vi "Spreadsheet String to Array Variant.vi"(8 "error in (no error)":errorcluster, 10 "spreadsheet string in":string, 11 "Array Variant in (type)":variant) -> (0 "error out":errorcluster, 3 "Array Variant out":variant)   [LabVIEW 2020, in "Generic Config Handling.lvlib"]
doc: "This vi converts a spreadsheet string into a variant which represents an array. The variant in is used to get the type."
uses:
  Generic Config Handling.lvlib
  <vilib>/Utility/VariantDataType/VariantType.lvlib
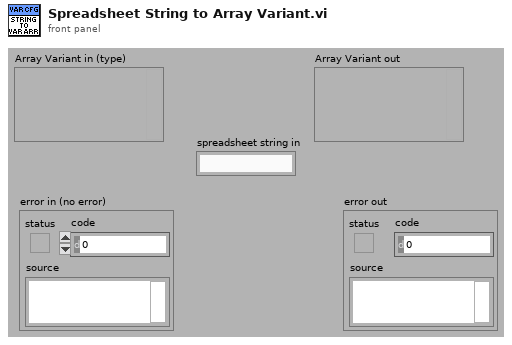
[diagram p1: front panel]
types:
  T1 = typedef "VariantType.lvlib/Type.ctl" = enum8{"Invalid Type", "Void", "I8", "I16", "I32", "I64", "U8", "U16", "U32", "U64", "Single Float", "Double Float", "Extended Float", "Single Complex", "Double Complex", "Extended Complex", "Enum U8", "Enum U16", "Enum U32", "Enum U64", "Single Float With Unit", "Double Float With Unit", "Extended Float With Unit", "Single Complex with Unit", "Double Complex with Unit", "Extended Complex with Unit", "Boolean", "String", "Path", "Picture", "Tag", "Array", "Cluster", "Variant", "LV Variant", "Waveform", "Timestamp", "Digital Waveform", "Digital Data", "ExpressData", "Refnum", "External Data", "VI", "Poly VI", "LabVIEW Class Instance", "Fixed Point"}
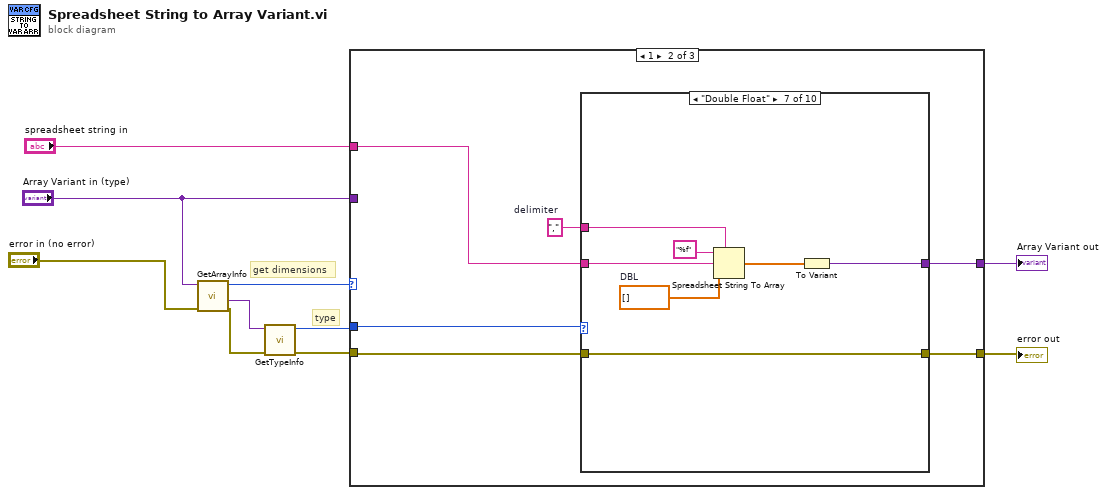
[diagram p0: block diagram]
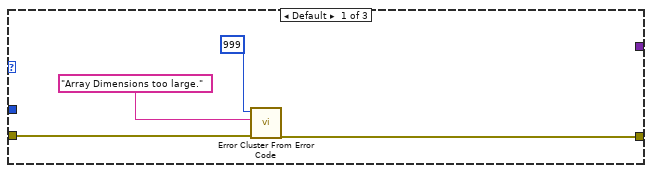
[diagram p2: hidden frame]
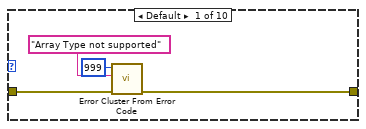
[diagram p3: hidden frame]
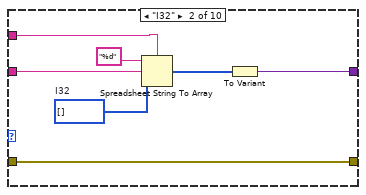
[diagram p4: hidden frame]
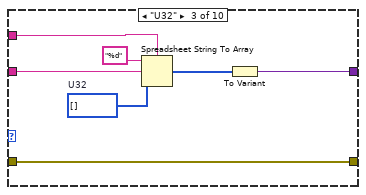
[diagram p5: hidden frame]
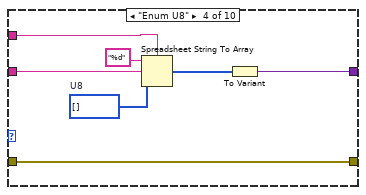
[diagram p6: hidden frame]
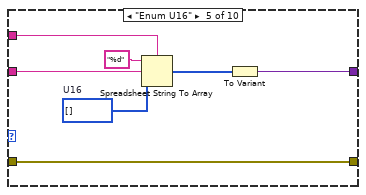
[diagram p7: hidden frame]
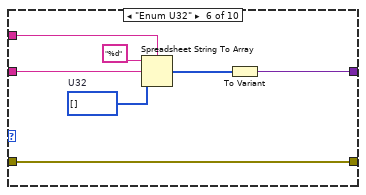
[diagram p8: hidden frame]
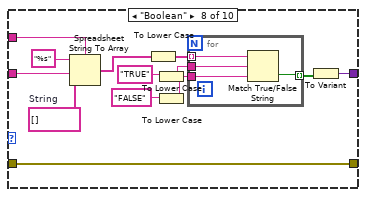
[diagram p9: hidden frame]
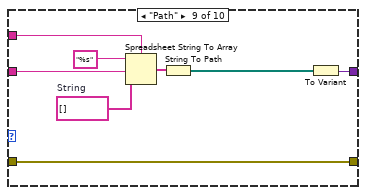
[diagram p10: hidden frame]
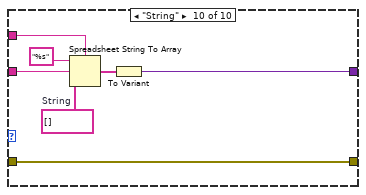
[diagram p11: hidden frame]
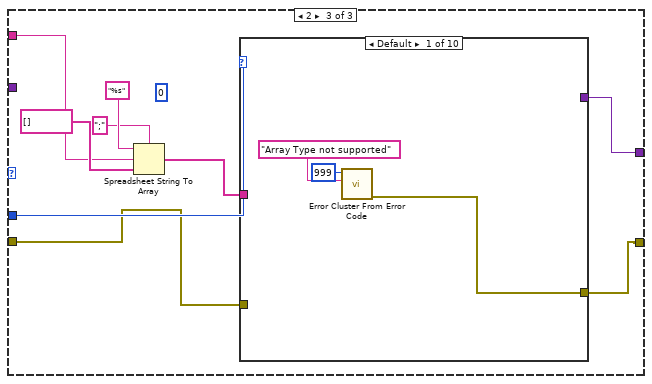
[diagram p12: hidden frame]
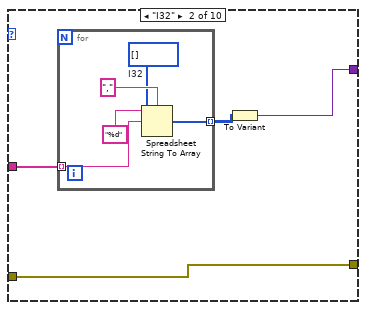
[diagram p13: hidden frame]
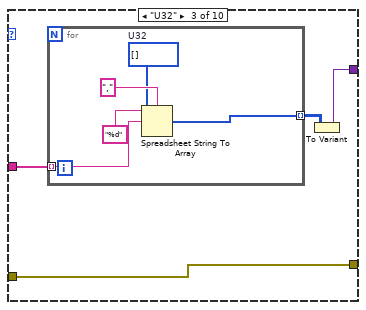
[diagram p14: hidden frame]
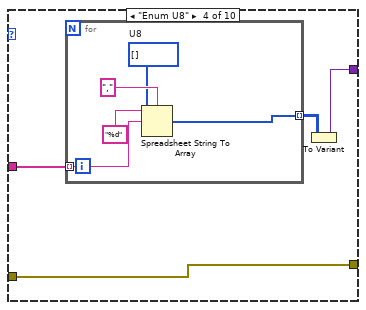
[diagram p15: hidden frame]
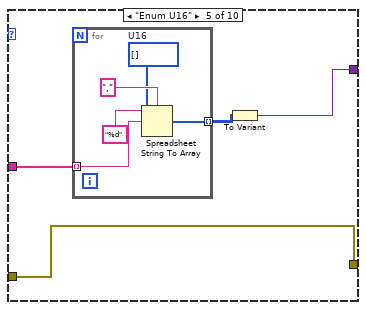
[diagram p16: hidden frame]
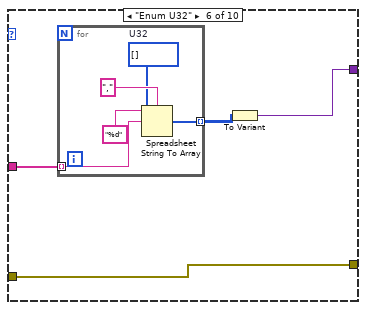
[diagram p17: hidden frame]
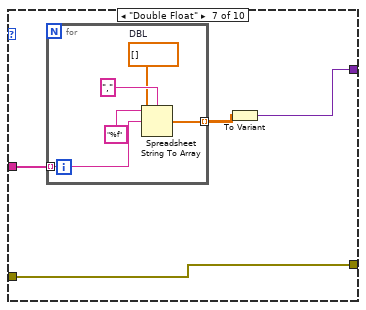
[diagram p18: hidden frame]
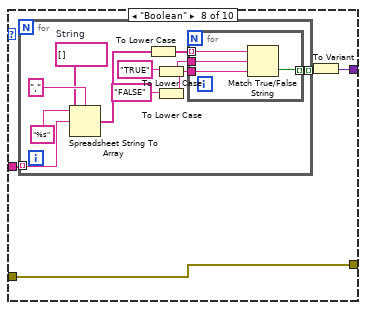
[diagram p19: hidden frame]
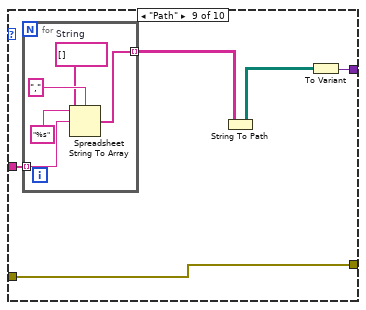
[diagram p20: hidden frame]
diagram:
  # "type"
  # "get dimensions"
  n1 = call <vilib>:"GetArrayInfo.vi"("error in (no error)"="error in (no error)", "Variant"="Array Variant in (type)") -> ("error out"=w7:errorcluster, "ArrayElement"=w6:variant, "NDims"=w4:i32)  [unwired: 6 in, 1 out]
  n2 = call <vilib>:"GetTypeInfo.vi"("error in (no error)"=w7, "Variant"=w6) -> ("error out"=w10:errorcluster, "Type Enum"=w8:T1)  [unwired: 5 in, 3 out]
  n3 = case shown="1" w4 {
    tunnel: w10 -> [w12 w18 w105]
    tunnel: [w11 w19 w106] -> w3
    tunnel: "Array Variant in (type)" -> [_ _ _]
    tunnel: w8 -> [_ w20 w107]
    tunnel: "spreadsheet string in" -> [_ w17 w100]
    tunnel: [_ w16 w104] -> w1
    frame Default {
      n4 = call <vilib>:"Error Cluster From Error Code.vi"("error in (no error)"=w12, "error message (\"\")"="Array Dimensions too large." ("error message (\"\")"), "error code (0)"=999) -> ("error out"=w11:errorcluster)  [unwired: 6 in]
    }
    frame 1 {
      w15 = ","  # delimiter
      n5 = case shown="\"Double Float\"" w20 {
        tunnel: [w22 w26 w33 w40 w47 w54 w61 w75 w87 w94] -> w19
        tunnel: w18 -> [w21 w26 w33 w40 w47 w54 w61 w75 w87 w94]
        tunnel: w17 -> [_ w31 w38 w45 w52 w59 w66 w79 w91 w98]
        tunnel: [_ w27 w34 w41 w48 w55 w62 w76 w88 w95] -> w16
        tunnel: w15 -> [_ w25 w32 w39 w46 w53 w60 w67 w84 w92]
        frame Default {
          n6 = call <vilib>:"Error Cluster From Error Code.vi"("error in (no error)"=w21, "error message (\"\")"="Array Type not supported" ("error message (\"\")"), "error code (0)"=999) -> ("error out"=w22:errorcluster)  [unwired: 6 in]
        }
        frame "I32" {
          w29 = i32[] []  # I32
          n7 = Spreadsheet String To Array(delimiter (Tab)=w25, format string="%d", spreadsheet string=w31, array type (2D Dbl)=w29) -> (array=w28:i32[])
          n8 = To Variant(anything=w28) -> (Variant=w27:variant)
        }
        frame "U32" {
          w36 = u32[] []  # U32
          n9 = Spreadsheet String To Array(delimiter (Tab)=w32, format string="%d", spreadsheet string=w38, array type (2D Dbl)=w36) -> (array=w35:u32[])
          n10 = To Variant(anything=w35) -> (Variant=w34:variant)
        }
        frame "Enum U8" {
          w43 = u8[] []  # U8
          n11 = Spreadsheet String To Array(delimiter (Tab)=w39, format string="%d", spreadsheet string=w45, array type (2D Dbl)=w43) -> (array=w42:u8[])
          n12 = To Variant(anything=w42) -> (Variant=w41:variant)
        }
        frame "Enum U16" {
          w50 = u16[] []  # U16
          n13 = Spreadsheet String To Array(delimiter (Tab)=w46, format string="%d", spreadsheet string=w52, array type (2D Dbl)=w50) -> (array=w49:u16[])
          n14 = To Variant(anything=w49) -> (Variant=w48:variant)
        }
        frame "Enum U32" {
          w57 = u32[] []  # U32
          n15 = Spreadsheet String To Array(delimiter (Tab)=w53, format string="%d", spreadsheet string=w59, array type (2D Dbl)=w57) -> (array=w56:u32[])
          n16 = To Variant(anything=w56) -> (Variant=w55:variant)
        }
        frame "Double Float" {
          w64 = dbl[] []  # DBL
          n17 = Spreadsheet String To Array(delimiter (Tab)=w60, format string="%f", spreadsheet string=w66, array type (2D Dbl)=w64) -> (array=w63:dbl[])
          n18 = To Variant(anything=w63) -> (Variant=w62:variant)
        }
        frame "Boolean" {
          w77 = string[] []  # String
          n19 = Spreadsheet String To Array(delimiter (Tab)=w67, format string="%s", spreadsheet string=w79, array type (2D Dbl)=w77) -> (array=w69:string[])
          n20 = To Lower Case(string=w69) -> (all lower case string=w74:string[])
          n21 = To Lower Case(string="TRUE" ("true string")) -> (all lower case string=w70:string)
          n22 = To Lower Case(string="FALSE" ("false string")) -> (all lower case string=w71:string)
          n23 = for {
            tunnel: w74 -> [w83] mode=indexing
            tunnel: w71 -> [w82]
            tunnel: w70 -> [w81]
            tunnel: [w80] -> w68 mode=indexing
            n24 = Match True/False String(2:w82, 3:w81, 4:w83) -> (0:w80:bool)  [unwired: 1 out]
          }
          n25 = To Variant(anything=w68) -> (Variant=w76:variant)
        }
        frame "Path" {
          w89 = string[] []  # String
          n26 = Spreadsheet String To Array(delimiter (Tab)=w84, format string="%s", spreadsheet string=w91, array type (2D Dbl)=w89) -> (array=w85:string[])
          n27 = String To Path(string=w85) -> (path=w86:path[])
          n28 = To Variant(anything=w86) -> (Variant=w88:variant)
        }
        frame "String" {
          w96 = string[] []  # String
          n29 = Spreadsheet String To Array(delimiter (Tab)=w92, format string="%s", spreadsheet string=w98, array type (2D Dbl)=w96) -> (array=w93:string[])
          n30 = To Variant(anything=w93) -> (Variant=w95:variant)
        }
      }
    }
    frame 2 {
      (unwired) u16 0
      n31 = Spreadsheet String To Array(delimiter (Tab)=";", format string="%s", spreadsheet string=w100, array type (2D Dbl)=string[] []) -> (array=w99:string[])
      n32 = case shown="Default" w107 {
        tunnel: [w108 w111 w122 w131 w138 w147 w156 w166 w186 w195] -> w106
        tunnel: w105 -> [_ w111 w122 w131 w138 w147 w156 w166 w186 w195]
        tunnel: w99 -> [_ w114 w123 w132 w141 w150 w159 w168 w188 w197]
        tunnel: [_ w112 w120 w129 w139 w148 w157 w167 w187 w196] -> w104
        frame Default {
          n33 = call <vilib>:"Error Cluster From Error Code.vi"("error message (\"\")"="Array Type not supported" ("error message (\"\")"), "error code (0)"=999) -> ("error out"=w108:errorcluster)  [unwired: 7 in]
        }
        frame "I32" {
          n34 = for {
            tunnel: w114 -> [w119] mode=indexing
            tunnel: [w115] -> w113 mode=indexing
            w116 = i32[] []  # I32
            n35 = Spreadsheet String To Array(delimiter (Tab)=",", format string="%d", spreadsheet string=w119, array type (2D Dbl)=w116) -> (array=w115:i32[])
          }
          n36 = To Variant(anything=w113) -> (Variant=w112:variant)
        }
        frame "U32" {
          n37 = for {
            tunnel: w123 -> [w128] mode=indexing
            tunnel: [w124] -> w121 mode=indexing
            w125 = u32[] []  # U32
            n38 = Spreadsheet String To Array(delimiter (Tab)=",", format string="%d", spreadsheet string=w128, array type (2D Dbl)=w125) -> (array=w124:u32[])
          }
          n39 = To Variant(anything=w121) -> (Variant=w120:variant)
        }
        frame "Enum U8" {
          n40 = for {
            tunnel: w132 -> [w137] mode=indexing
            tunnel: [w133] -> w130 mode=indexing
            w134 = u8[] []  # U8
            n41 = Spreadsheet String To Array(delimiter (Tab)=",", format string="%d", spreadsheet string=w137, array type (2D Dbl)=w134) -> (array=w133:u8[])
          }
          n42 = To Variant(anything=w130) -> (Variant=w129:variant)
        }
        frame "Enum U16" {
          n43 = for {
            tunnel: w141 -> [w146] mode=indexing
            tunnel: [w142] -> w140 mode=indexing
            w143 = u16[] []  # U16
            n44 = Spreadsheet String To Array(delimiter (Tab)=",", format string="%d", spreadsheet string=w146, array type (2D Dbl)=w143) -> (array=w142:u16[])
          }
          n45 = To Variant(anything=w140) -> (Variant=w139:variant)
        }
        frame "Enum U32" {
          n46 = for {
            tunnel: w150 -> [w155] mode=indexing
            tunnel: [w151] -> w149 mode=indexing
            w152 = u32[] []  # U32
            n47 = Spreadsheet String To Array(delimiter (Tab)=",", format string="%d", spreadsheet string=w155, array type (2D Dbl)=w152) -> (array=w151:u32[])
          }
          n48 = To Variant(anything=w149) -> (Variant=w148:variant)
        }
        frame "Double Float" {
          n49 = for {
            tunnel: w159 -> [w164] mode=indexing
            tunnel: [w160] -> w158 mode=indexing
            w161 = dbl[] []  # DBL
            n50 = Spreadsheet String To Array(delimiter (Tab)=",", format string="%f", spreadsheet string=w164, array type (2D Dbl)=w161) -> (array=w160:dbl[])
          }
          n51 = To Variant(anything=w158) -> (Variant=w157:variant)
        }
        frame "Boolean" {
          n52 = for {
            tunnel: w168 -> [w179] mode=indexing
            tunnel: [w169] -> w165 mode=indexing
            w176 = string[] []  # String
            n53 = Spreadsheet String To Array(delimiter (Tab)=",", format string="%s", spreadsheet string=w179, array type (2D Dbl)=w176) -> (array=w170:string[])
            n54 = To Lower Case(string=w170) -> (all lower case string=w175:string[])
            n55 = To Lower Case(string="TRUE" ("true string")) -> (all lower case string=w171:string)
            n56 = To Lower Case(string="FALSE" ("false string")) -> (all lower case string=w172:string)
            n57 = for {
              tunnel: w175 -> [w183] mode=indexing
              tunnel: w172 -> [w182]
              tunnel: w171 -> [w181]
              tunnel: [w180] -> w169 mode=indexing
              n58 = Match True/False String(2:w182, 3:w181, 4:w183) -> (0:w180:bool)  [unwired: 1 out]
            }
          }
          n59 = To Variant(anything=w165) -> (Variant=w167:variant)
        }
        frame "Path" {
          n60 = for {
            tunnel: w188 -> [w193] mode=indexing
            tunnel: [w189] -> w185 mode=indexing
            w190 = string[] []  # String
            n61 = Spreadsheet String To Array(delimiter (Tab)=",", format string="%s", spreadsheet string=w193, array type (2D Dbl)=w190) -> (array=w189:string[])
          }
          n62 = String To Path(string=w185) -> (path=w184:path[][])
          n63 = To Variant(anything=w184) -> (Variant=w187:variant)
        }
        frame "String" {
          n64 = for {
            tunnel: w197 -> [w202] mode=indexing
            tunnel: [w198] -> w194 mode=indexing
            w199 = string[] []  # String
            n65 = Spreadsheet String To Array(delimiter (Tab)=",", format string="%s", spreadsheet string=w202, array type (2D Dbl)=w199) -> (array=w198:string[])
          }
          n66 = To Variant(anything=w194) -> (Variant=w196:variant)
        }
      }
    }
  }
  "error out" <- w3
  "Array Variant out" <- w1
